vi "RC_Circuits.vi"() -> ()   [LabVIEW 2022 SP3]
panel:
  in  "Time (s)":i32=125
  out "Vc (V)":dbl format="%#_13g"
  # "RC_Circuits:\nFor an RC Circuit with the following configuration,\n    Vs = 12V\n    R = 0.5 ohms\n    C = 1e-6 Farads\nEnter a value for time to see the voltage across the \ncapacitor during a charging cycle."
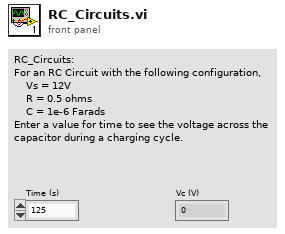
[diagram p1: front panel]
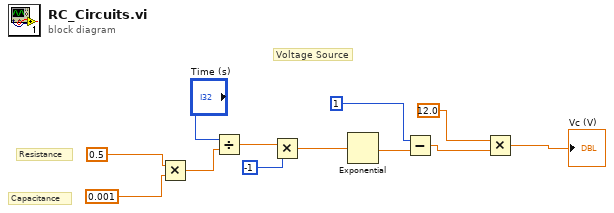
[diagram p0: block diagram]
diagram:
  # "Voltage Source"
  # "Capacitance"
  # "Resistance"
  n1 = Multiply(x=0.5, y=0.001) -> (x*y=w9:dbl)
  n2 = Divide(x="Time (s)", y=w9) -> (x/y=w8:dbl)
  n3 = Multiply(x=w8, y=-1) -> (x*y=w7:dbl)
  n4 = Exponential(1:w7) -> (0:w3:dbl)
  n5 = Subtract(x=1, y=w3) -> (x-y=w1:dbl)
  n6 = Multiply(x=12.0, y=w1) -> (x*y=→"Vc (V)":dbl)
